vi "DFD Convert Integer to FXP.vi"   [LabVIEW 2017, in "NI_DigFilterLicensed.lvlib"]
doc: "Converts integers to fixed-point numbers. Wire data to the <B>I16</B> input to determine the polymorphic instance to use or manually select the instance."
uses:
  <vilib>/addons/Digital Filter Design/NI_DigFilterLicensed.lvlib
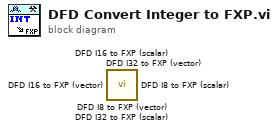
[diagram p0: block diagram]
diagram:
  n1 = call <vilib>:"DFD I8 to FXP (vector).vi"() -> ()  [unwired: 10 in, 2 out]
  n2 = call <vilib>:"DFD I32 to FXP (vector).vi"() -> ()  [unwired: 10 in, 2 out]
  n3 = call <vilib>:"DFD I16 to FXP (vector).vi"() -> ()  [unwired: 10 in, 2 out]
  n4 = call <vilib>:"DFD I8 to FXP (scalar).vi"() -> ()  [unwired: 10 in, 2 out]
  n5 = call <vilib>:"DFD I32 to FXP (scalar).vi"() -> ()  [unwired: 10 in, 2 out]
  n6 = call <vilib>:"DFD I16 to FXP (scalar).vi"() -> ()  [unwired: 10 in, 2 out]
